vi "1820 Build.vi"() -> ()   [LabVIEW 2019]
uses:
  <vilib>/AppBuilder/AB_API_Simple/Build Specification Version.ctl
  <vilib>/AppBuilder/AB_API_Simple/Set Build Specification Version (path).vi
  <vilib>/AppBuilder/AB_API_Simple/Build (path).vi
  <userlib>/LevyLab/Build Support/PostBuildSupport/PostBuildSupport.lvclass
  <vilib>/MakerHub/Toolbox/LMH-Toolbox.lvlib
  <vilib>/AppBuilder/AB_API_Simple/NI_App_Builder_API.lvlib
panel:
  in  "Package Version (maj.min.fix.build)":string="1.3.2.21"
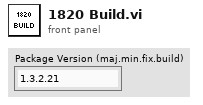
[diagram p1: front panel]
types:
  T1 = typedef "NI_App_Builder_API.lvlib/Build Specification Version.ctl" = cluster{"Major":u16, "Minor":u16, "Fix":u16, "Build":u16}
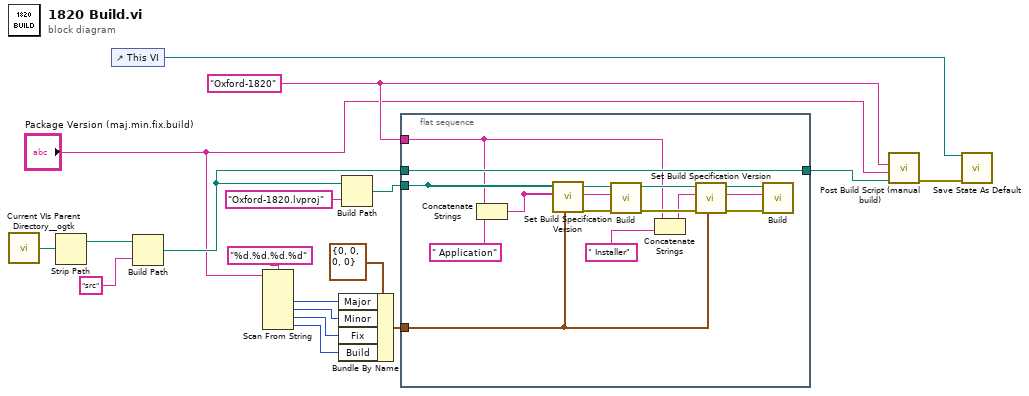
[diagram p0: block diagram]
diagram:
  w4 = "Oxford-1820" ("Product Name")
  n1 = call <userlib>:"Current VIs Parent Directory__ogtk.vi"() -> ("Parent Directory (+ Relative)"=w18:path)  [unwired: 5 in]
  n2 = Strip Path(path=w18) -> (stripped path=w17:path)  [unwired: 1 out]
  n3 = control-ref of="This VI"() -> (w14:refnum<vi>)
  n4 = Build Path(base path=w17, name or relative path="src") -> (appended path=w3:path)
  n5 = Scan From String(format string="%d.%d.%d.%d", input string="Package Version (maj.min.fix.build)") -> (output 1=w10:i32, output 2=w13:i32, output 3=w9:i32, output 4=w12:i32)  [unwired: 6 in, 3 out]
  n6 = Bundle By Name(cluster=T1 {"Major"=0, "Minor"=0, "Fix"=0, "Build"=0} ("Build Specification Version"), "Major"=w10, "Minor"=w13, "Fix"=w9, "Build"=w12) -> (w7:T1)
  n7 = Build Path(base path=w3, name or relative path="Oxford-1820.lvproj") -> (appended path=w5:path)
  n8 = flat-sequence {
    tunnel: w7 -> [w27]
    tunnel: w5 -> [w25]
    tunnel: [w24] -> w2
    tunnel: w3 -> [w24]
    tunnel: w4 -> [w20]
    frame #0 {
      n9 = Concatenate Strings(w20, " Application" ("Name of build specification")) -> (w22:string)
      n10 = call-poly <vilib>:"Set Build Specification Version.vi"("Build Specification Version"=w27, "Name of build specification"=w22, "Path to project"=w25) -> ("error out"=w29:errorcluster)  [unwired: 8 in]
      n11 = call-poly <vilib>:"Build.vi"("error in (no error)"=w29, "Name of build specification (if empty: build all)"=w22, "Path to project"=w25) -> ("error out"=w28:errorcluster)  [unwired: 7 in, 1 out]
      n12 = Concatenate Strings(w20, " Installer" ("Name of build specification")) -> (w19:string)
      n13 = call-poly <vilib>:"Set Build Specification Version.vi"("Build Specification Version"=w27, "error in (no error)"=w28, "Name of build specification"=w19, "Path to project"=w25) -> ("error out"=w26:errorcluster)  [unwired: 7 in]
      n14 = call-poly <vilib>:"Build.vi"("error in (no error)"=w26, "Name of build specification (if empty: build all)"=w19, "Path to project"=w25) -> ()  [unwired: 7 in, 2 out]
    }
  }
  n15 = call <userlib>:"Post Build Script (manual build).vi"("Package Source Folder"=w2, "Package Version"="Package Version (maj.min.fix.build)", "Product Name"=w4) -> ("error out"=w15:errorcluster)  [unwired: 8 in]
  n16 = call <vilib>:"Save State As Default.vi"("Error In"=w15, "Target VI"=w14) -> ()  [unwired: 8 in, 2 out]
